vi "Create Sysdef Tree from Parameters Clusters_Find Label Refs.vi"(0 "Item Ref in":T1 format="%.0x", 5 "decimalLabel":i32, 7 "SDI_Enabled":bool, 9 "SDIValue":u8, 11 "error in (no error)":errorcluster) -> (4 "Array of Refs":T1[](array[typedef]) format="%.0x", 6 "Found":bool, 15 "error out":errorcluster)   [LabVIEW 2016, in "Ballard Arinc-429 System Explorer.lvlib"]
uses:
  Ballard Arinc-429 System Explorer.lvlib
  <vilib>/NI Veristand/Custom Device API/Custom Device Item Ref.ctl
  <vilib>/NI Veristand/Custom Device API/Get Item Property (U32).vi
  Shared/Controls and Global/Global.vi
  <vilib>/NI Veristand/Custom Device API/Get Item Property (Boolean).vi
  <vilib>/NI VeriStand/Custom Device API/Custom Device API.lvlib
  Shared/Ballard Arinc-429 Shared.lvlib
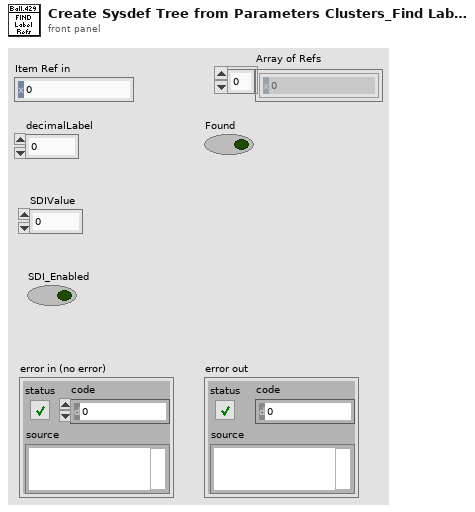
[diagram p1: front panel]
types:
  T1 = typedef "Custom Device API.lvlib/Custom Device Item Ref.ctl" = u64
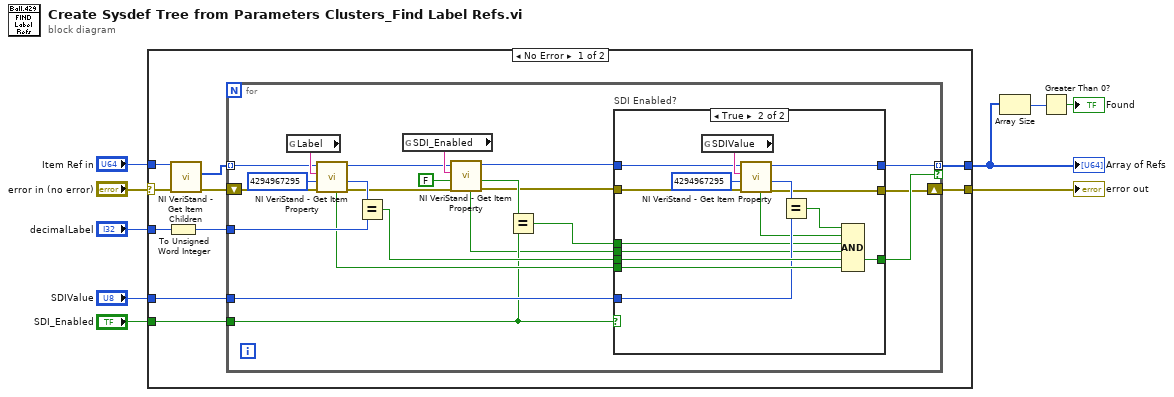
[diagram p0: block diagram]
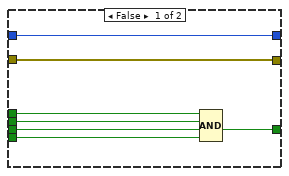
[diagram p2: hidden frame]
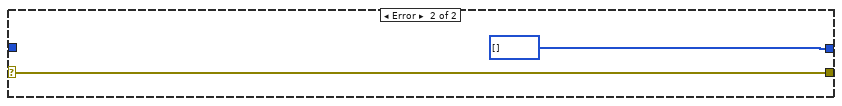
[diagram p3: hidden frame]
diagram:
  n1 = case shown="No Error" "error in (no error)" {
    selector: "error in (no error)" -> [w15 w65]
    tunnel: "decimalLabel" -> [w19 _]
    tunnel: [w18 w65] -> w8
    tunnel: "Item Ref in" -> [w17 _]
    tunnel: [w12 T1[] [] ("Array of Refs")] -> w5
    tunnel: "SDIValue" -> [w11 _]
    tunnel: "SDI_Enabled" -> [w10 _]
    frame No Error {
      n2 = To Unsigned Word Integer(number=w19) -> (unsigned 16bit integer=w14:u16)
      n3 = call <vilib>:"NI VeriStand - Get Item Children.vi"("error in (no error)"=w15, "Item Ref in"=w17) -> ("error out"=w16:errorcluster, "Child Refs"=w13:T1[])  [unwired: 6 in, 2 out]
      n4 = for {
        tunnel: w14 -> [w40]
        shift-right: [w30] -> w18
        shift-left: w16 -> [w41]
        tunnel: w13 -> [w36] mode=indexing
        tunnel: [w34] -> w12 mode=indexing if=w35
        tunnel: w11 -> [w31]
        tunnel: w10 -> [w24]
        n5 = global read "Global.vi" "Label"() -> (w38:string)
        n6 = call-poly <vilib>:"NI VeriStand - Get Item Property.vi"("error in (no error)"=w41, "Default Value"=u32 4294967295, "Property Name"=w38, "Item Ref in"=w36) -> ("error out"=w23:errorcluster, "Value"=w37:u32, "Item Ref out"=w26:T1, "Found?"=w32:bool)  [unwired: 4 in]
        n7 = Equal?(x=w37, y=w40) -> (x = y?=w33:bool)
        n8 = global read "Global.vi" "SDI_Enabled"() -> (w28:string)
        n9 = call-poly <vilib>:"NI VeriStand - Get Item Property.vi"("error in (no error)"=w23, "Default Value"=FALSE, "Property Name"=w28, "Item Ref in"=w26) -> ("error out"=w22:errorcluster, "Value"=w27:bool, "Item Ref out"=w25:T1, "Found?"=w21:bool)  [unwired: 4 in]
        n10 = Equal?(x=w27, y=w24) -> (x = y?=w20:bool)
        n11 = case "SDI Enabled?" shown="True" w24 {
          tunnel: [w46 w63] -> w35
          tunnel: w25 -> [w48 w59]
          tunnel: [w48 w58] -> w34
          tunnel: w33 -> [w45 w57]
          tunnel: w32 -> [w44 w56]
          tunnel: w31 -> [_ w55]
          tunnel: w22 -> [w47 w54]
          tunnel: [w47 w53] -> w30
          tunnel: w21 -> [w43 w52]
          tunnel: w20 -> [w42 w51]
          frame False {
            n12 = Compound Arithmetic op=AND(w42, w43, w45, w44) -> (w46:bool)
          }
          frame True {
            n13 = global read "Global.vi" "SDIValue"() -> (w61:string)
            n14 = call-poly <vilib>:"NI VeriStand - Get Item Property.vi"("error in (no error)"=w54, "Default Value"=u32 4294967295, "Property Name"=w61, "Item Ref in"=w59) -> ("error out"=w53:errorcluster, "Value"=w62:u32, "Item Ref out"=w58:T1, "Found?"=w50:bool)  [unwired: 4 in]
            n15 = Equal?(x=w62, y=w55) -> (x = y?=w49:bool)
            n16 = Compound Arithmetic op=AND(w49, w50, w51, w52, w57, w56) -> (w63:bool)
          }
        }
      }
    }
    frame Error {
    }
  }
  "error out" <- w8
  "Array of Refs" <- w5
  n17 = Array Size(array=w5) -> (size(s)=w4:i32)
  n18 = Greater Than 0?(x=w4) -> (x > 0?=→"Found":bool)
